vi "multi_enent_data_queues.vi"(6 "Front?":bool, 7 "Mode":T2, 8 "error in":errorcluster, 9 "data":cluster{"Time Stamp":timestamp, "data":string}, 10 "process":cluster{"event":string, "Message":string}, 11 "name":string) -> (0 "error out":errorcluster, 1 "data 2":cluster{"time":timestamp, "data":string}, 2 "process":cluster{"event":string, "par":string}, 3 "timed out?":bool, 4 "remaining elements":cluster{"time":timestamp, "data":string}[](array[cluster]))   [LabVIEW 2015]
uses:
  multi_queue_enum.ctl
panel:
  in  "queues":T1
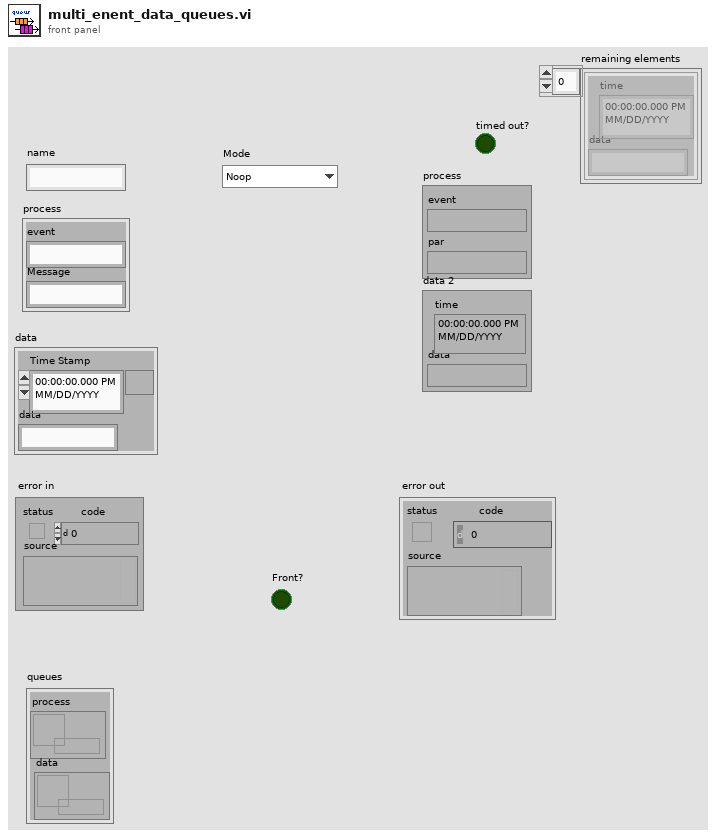
[diagram p1: front panel]
types:
  T1 = cluster{"process":refnum<queue>, "data":refnum<queue>}
  T2 = typedef "multi_queue_enum.ctl" = enum16{"Noop", "add queues", "Send Pro1", "Send data", "Get Pro1", "Get data", "Flush Pro1", "Flush data", "Destroy Pro1", "Destroy data"}
  T3 = cluster{"process":refnum<queue>, "data":refnum<queue>}[]
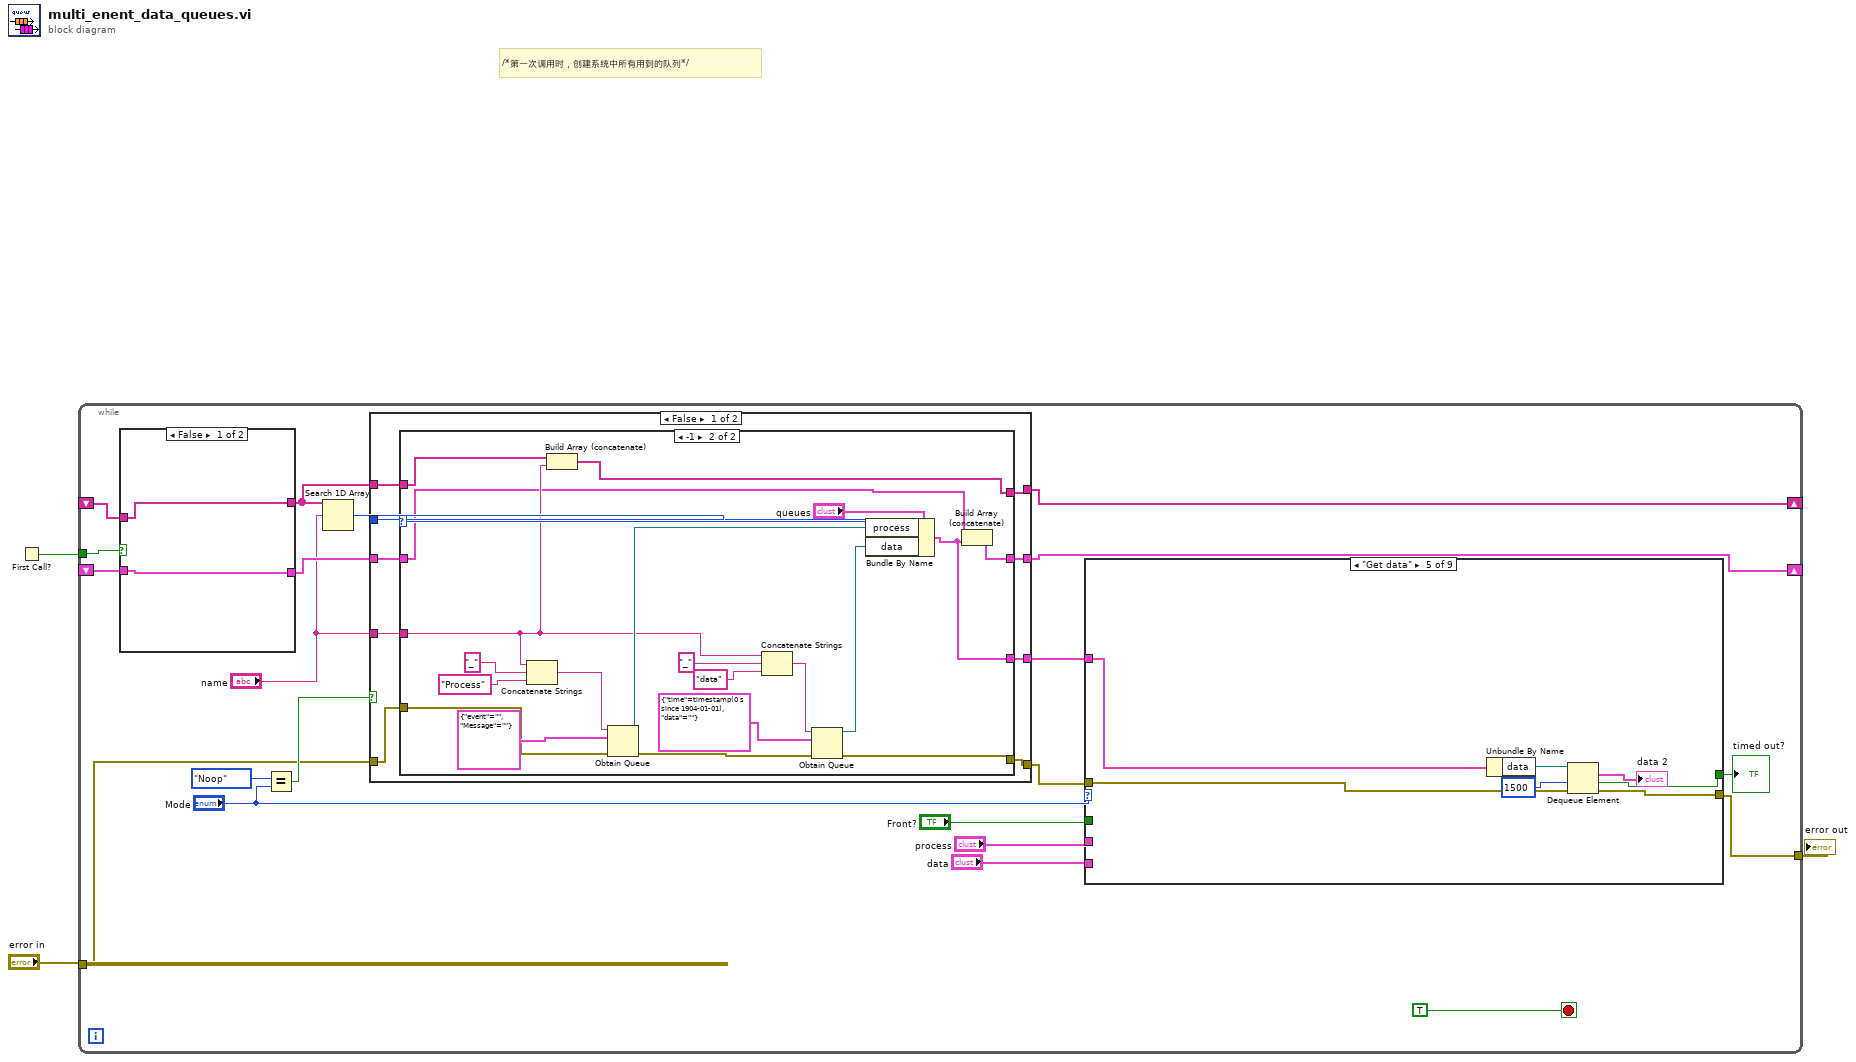
[diagram p0: block diagram]
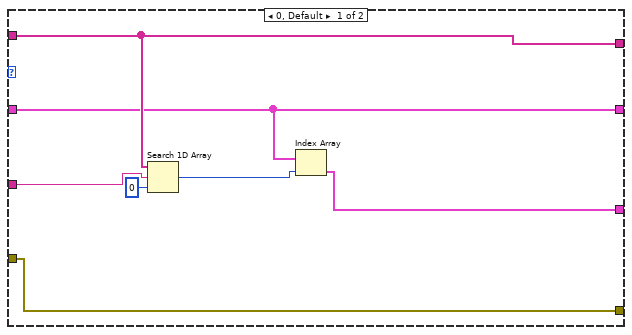
[diagram p2: hidden frame]
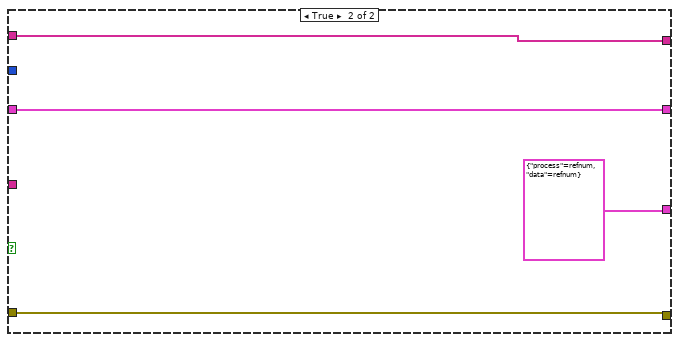
[diagram p3: hidden frame]
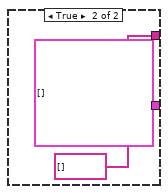
[diagram p4: hidden frame]
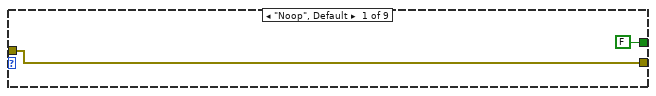
[diagram p5: hidden frame]
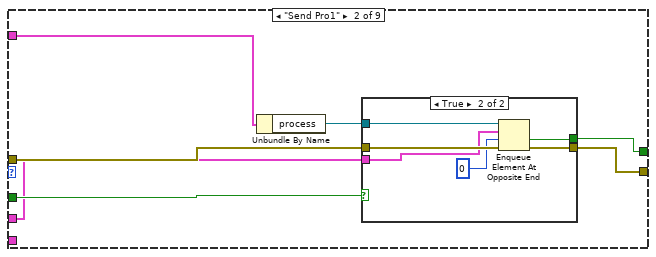
[diagram p6: hidden frame]
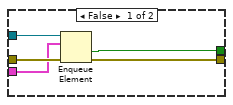
[diagram p7: hidden frame]
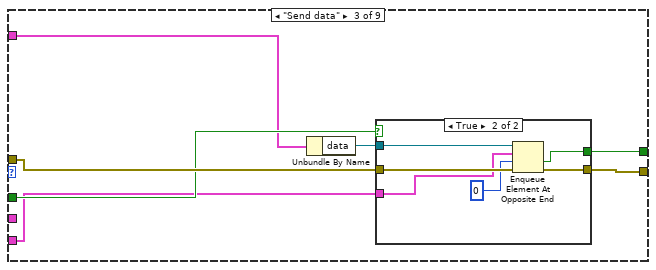
[diagram p8: hidden frame]
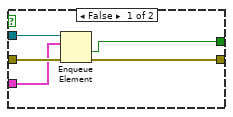
[diagram p9: hidden frame]
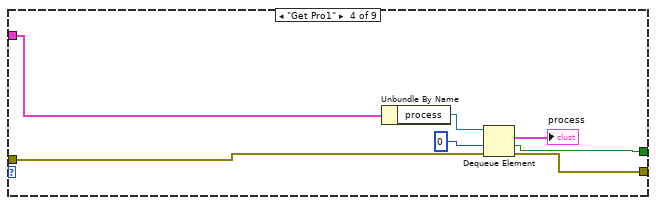
[diagram p10: hidden frame]
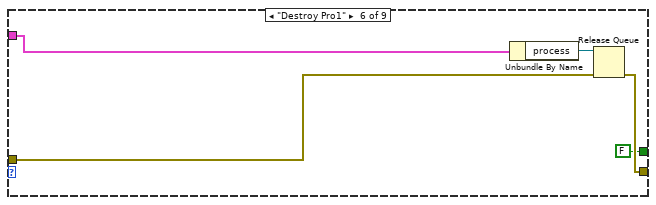
[diagram p11: hidden frame]
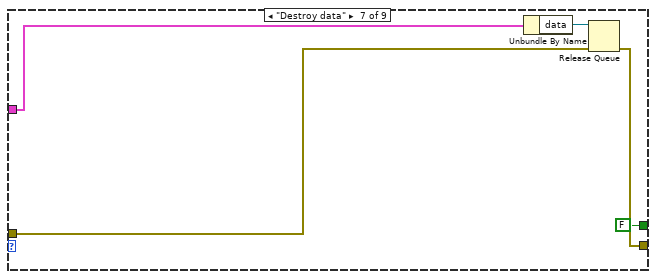
[diagram p12: hidden frame]
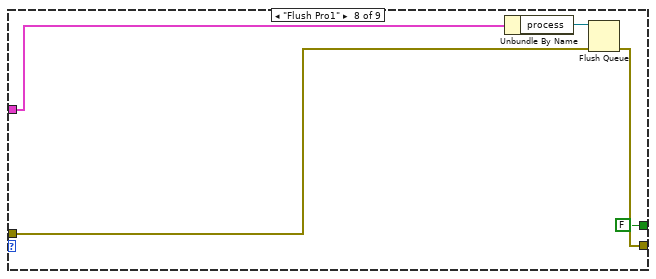
[diagram p13: hidden frame]
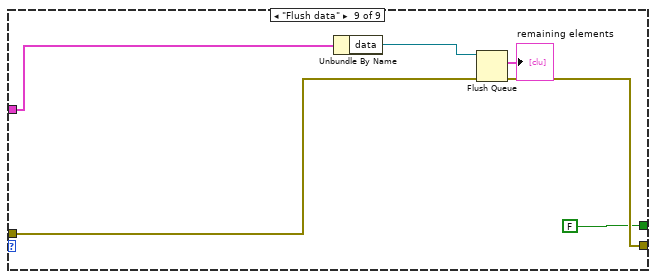
[diagram p14: hidden frame]
diagram:
  # "/*第一次调用时，创建系统中所有用到的队列*/"
  n1 = First Call?() -> (First Call?: T/F=w3:bool)
  n2 = while {
    tunnel: w3 -> [w22]
    tunnel: [w10] -> w1
    shift-right: [w7] -> _
    shift-left: _ -> [w21]
    tunnel: "error in" -> [w11]
    shift-right: [w8] -> _
    shift-left: _ -> [w20]
    stop <- TRUE stop-if-true
    n3 = case shown="False" w22 {
      tunnel: [w66 T3 []] -> w17
      tunnel: [w65 string[] []] -> w18
      tunnel: w21 -> [w66 _]
      tunnel: w20 -> [w65 _]
      frame False {
      }
      frame True {
      }
    }
    n4 = Equal?(x=multi_queue_enum."Noop", y="Mode") -> (x = y?=w15:bool)
    n5 = Search 1D Array(1D array=w18, element="name") -> (index of element=w19:i32)  [unwired: 1 in]
    n6 = case shown="False" w15 {
      tunnel: w19 -> [w33 _]
      tunnel: w18 -> [w32 w64]
      tunnel: [w31 w64] -> w8
      tunnel: w17 -> [w30 w63]
      tunnel: [w29 w63] -> w7
      tunnel: "name" -> [w28 _]
      tunnel: w11 -> [w27 w61]
      tunnel: [w26 w61] -> w12
      tunnel: [w25 T1 {"process"=refnum, "data"=refnum} ("queues")] -> w9
      frame False {
        n7 = case shown="-1" w33 {
          tunnel: w32 -> [w39 w47]
          tunnel: [w39 w45] -> w31
          tunnel: w30 -> [w37 w44]
          tunnel: [w37 w48] -> w29
          tunnel: w28 -> [w38 w46]
          tunnel: w27 -> [w34 w43]
          tunnel: [w34 w42] -> w26
          tunnel: [w35 w41] -> w25
          frame 0, Default {
            n8 = Search 1D Array(1D array=w39, element=w38, start index (0)=0) -> (index of element=w36:i32)
            n9 = Index Array(array=w37, index=w36) -> (element=w35:T1)
          }
          frame -1 {
            n10 = Concatenate Strings(w46, "_" ("string"), "Process" ("name (unnamed)")) -> (w57:string)
            n11 = Build Array (concatenate)(w47, w46) -> (w45:string[])
            n12 = Obtain Queue(name (unnamed)=w57, element data type=cluster{"event":string, "Message":string} {"event"="", "Message"=""} ("Cluster"), error in (no error)=w43) -> (queue out=w50:refnum<queue>, error out=w51:errorcluster)  [unwired: 2 in, 1 out]
            n13 = Concatenate Strings(w46, "_" ("string"), "data") -> (w60:string)
            n14 = Obtain Queue(name (unnamed)=w60, element data type=cluster{"time":timestamp, "data":string} {"time"=timestamp(0 s since 1904-01-01), "data"=""} ("Cluster"), error in (no error)=w51) -> (queue out=w49:refnum<queue>, error out=w42:errorcluster)  [unwired: 2 in, 1 out]
            n15 = Bundle By Name(cluster="queues", "process"=w50, "data"=w49) -> (w41:T1)
            n16 = Build Array (concatenate)(w44, w41) -> (w48:T3)
          }
        }
      }
      frame True {
      }
    }
    n17 = case shown="\"Get data\"" "Mode" {
      tunnel: w12 -> [w70 w77 w95 w112 w119 w125 w130 w134 w140]
      tunnel: [w70 w76 w94 w111 w118 w124 w129 w133 w139] -> w10
      tunnel: "Front?" -> [_ w75 w93 _ _ _ _ _ _]
      tunnel: "process" -> [_ w73 _ _ _ _ _ _ _]
      tunnel: "data" -> [_ _ w91 _ _ _ _ _ _]
      tunnel: w9 -> [_ w72 w90 w108 w115 w122 w127 w132 w138]
      tunnel: [FALSE ("timed out?") w71 w89 w107 w114 FALSE ("timed out?") FALSE ("timed out?") FALSE ("timed out?") FALSE ("timed out?")] -> w4
      frame "Noop", Default {
      }
      frame "Send Pro1" {
        n18 = Unbundle By Name(w72) -> ("process"=w74:refnum<queue>)
        n19 = case shown="True" w75 {
          tunnel: w77 -> [w82 w88]
          tunnel: [w81 w87] -> w76
          tunnel: w74 -> [w80 w85]
          tunnel: w73 -> [w79 w84]
          tunnel: [w78 w83] -> w71
          frame False {
            n20 = Enqueue Element(queue=w80, element=w79, error in (no error)=w82) -> (timed out?=w78:bool, error out=w81:errorcluster)  [unwired: 2 out]
          }
          frame True {
            n21 = Enqueue Element At Opposite End(queue=w85, element=w84, timeout in ms (-1)=0, error in (no error)=w88) -> (timed out?=w83:bool, error out=w87:errorcluster)  [unwired: 1 out]
          }
        }
      }
      frame "Send data" {
        n22 = Unbundle By Name(w90) -> ("data"=w92:refnum<queue>)
        n23 = case shown="True" w93 {
          tunnel: w95 -> [w100 w106]
          tunnel: [w99 w105] -> w94
          tunnel: w92 -> [w98 w103]
          tunnel: w91 -> [w97 w102]
          tunnel: [w96 w101] -> w89
          frame False {
            n24 = Enqueue Element(queue=w98, element=w97, error in (no error)=w100) -> (timed out?=w96:bool, error out=w99:errorcluster)  [unwired: 1 in, 1 out]
          }
          frame True {
            n25 = Enqueue Element At Opposite End(queue=w103, element=w102, timeout in ms (-1)=0, error in (no error)=w106) -> (timed out?=w101:bool, error out=w105:errorcluster)  [unwired: 1 out]
          }
        }
      }
      frame "Get Pro1" {
        n26 = Unbundle By Name(w108) -> ("process"=w113:refnum<queue>)
        n27 = Dequeue Element(queue=w113, timeout in ms (-1)=0, error in (no error)=w112) -> (element=→"process":cluster{"event":string, "par":string}, timed out?=w107:bool, error out=w111:errorcluster)  [unwired: 1 out]
      }
      frame "Get data" {
        n28 = Unbundle By Name(w115) -> ("data"=w120:refnum<queue>)
        n29 = Dequeue Element(queue=w120, timeout in ms (-1)=1500, error in (no error)=w119) -> (element=→"data 2":cluster{"time":timestamp, "data":string}, timed out?=w114:bool, error out=w118:errorcluster)  [unwired: 1 out]
      }
      frame "Destroy Pro1" {
        n30 = Unbundle By Name(w122) -> ("process"=w123:refnum<queue>)
        n31 = Release Queue(queue=w123, error in (no error)=w125) -> (error out=w124:errorcluster)  [unwired: 3 out]
      }
      frame "Destroy data" {
        n32 = Unbundle By Name(w127) -> ("data"=w128:refnum<queue>)
        n33 = Release Queue(queue=w128, error in (no error)=w130) -> (error out=w129:errorcluster)  [unwired: 3 out]
      }
      frame "Flush Pro1" {
        n34 = Unbundle By Name(w132) -> ("process"=w135:refnum<queue>)
        n35 = Flush Queue(queue=w135, error in (no error)=w134) -> (error out=w133:errorcluster)  [unwired: 2 out]
      }
      frame "Flush data" {
        n36 = Unbundle By Name(w138) -> ("data"=w141:refnum<queue>)
        n37 = Flush Queue(queue=w141, error in (no error)=w140) -> (remaining elements=→"remaining elements":cluster{"time":timestamp, "data":string}[], error out=w139:errorcluster)  [unwired: 1 out]
      }
    }
    "timed out?" <- w4
  }
  "error out" <- w1
